vi "Export Configuration RTM.vi"(8 "error in":errorcluster, 11 "Node Ptr":u64 format="%.0x") -> (0 "error out":errorcluster)   [LabVIEW 2026, in "NIDMM System Explorer.lvlib"]
uses:
  NIDMM System Explorer.lvlib
  NationalInstruments.VeriStand.SystemDefinitionAPI
panel:
  in  "Tag":string
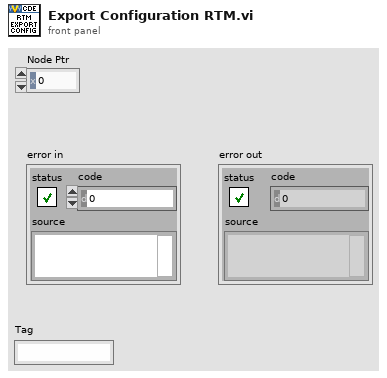
[diagram p1: front panel]
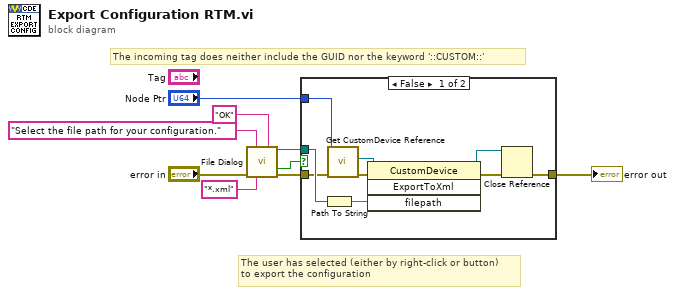
[diagram p0: block diagram]
diagram:
  # "The user has selected (either by right-click or button)\nto export the configuration"
  # "The incoming tag does neither include the GUID nor the keyword '::CUSTOM::'"
  n1 = call "File Dialog"("prompt"="Select the file path for your configuration.", "button label"="OK", "error in"="error in", "pattern (all files)"="*.xml") -> ("selected path"=w7:path, "cancelled"=w8:bool, "error out"=w9:errorcluster)  [unwired: 8 in, 1 out]
  n2 = case shown="False" w8 {
    tunnel: [w12 w19] -> w1
    tunnel: w9 -> [w15 w19]
    tunnel: w7 -> [w18 _]
    tunnel: "Node Ptr" -> [w10 _]
    frame False {
      n3 = Path To String(path=w18) -> (string=w11:string)
      n4 = call "Get CustomDevice Reference.vi"("error in"=w15, "Node Ptr"=w10) -> ("error out"=w14:errorcluster, "Custom Device"=w16:refnum<k24>)  [unwired: 7 in, 1 out]
      n5 = invoke class="CustomDevice" method="ExportToXml"(reference=w16, error in=w14, "filepath"=w11) -> (reference out=w17:refnum<k24>, error out=w13:errorcluster)  [unwired: 1 in, 2 out]
      n6 = Close Reference(reference=w17, error in (no error)=w13) -> (error out=w12:errorcluster)
    }
    frame True {
    }
  }
  "error out" <- w1
